vi "AndorError2MultiList.vi"(8 "error in (no error)":errorcluster, 11 "Errors Messages":cluster{i32, string}[](array[cluster])) -> (0 "error out":errorcluster, 3 "Array":string[][](array[string]))   [LabVIEW 2018, in "AndorOWN.lvlib"]
uses:
  AndorOWN.lvlib
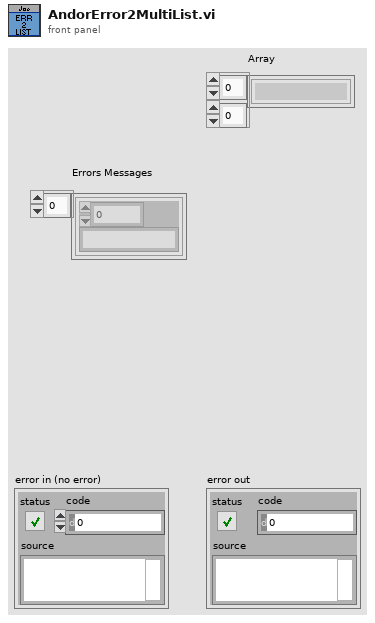
[diagram p1: front panel]
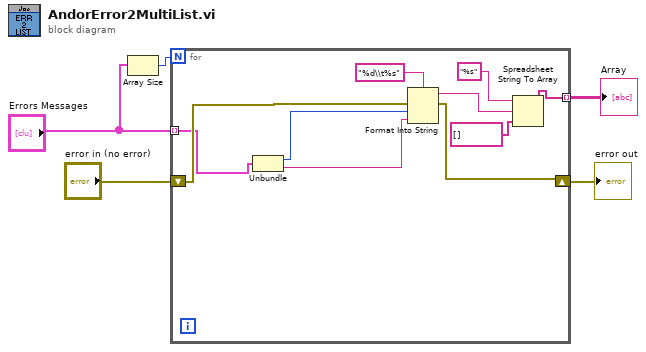
[diagram p0: block diagram]
diagram:
  n1 = Array Size(array="Errors Messages") -> (size(s)=w2:i32)
  n2 = for {
    N: w2 -> [_]
    tunnel: "Errors Messages" -> [w8] mode=indexing
    tunnel: [w10] -> w5 mode=indexing
    shift-right: [w13] -> w4
    shift-left: "error in (no error)" -> [w15]
    n3 = Unbundle(w8) -> (w7:i32, w6:string)
    n4 = Format Into String(format string="%d\\t%s", error in=w15, w7, w6) -> (resulting string=w12:string, error out=w13:errorcluster)  [unwired: 1 in]
    n5 = Spreadsheet String To Array(format string="%s", spreadsheet string=w12, array type (2D Dbl)=string[] []) -> (array=w10:string[])  [unwired: 1 in]
  }
  "Array" <- w5
  "error out" <- w4
